vi "Set Up Dialog - Goniometer .vi"() -> ()   [LabVIEW 2012]
panel:
  out "Calibration Instructions":string="1. Connect the sensor to your myDAQ as shown in the diagram above.\n\n2. Use a text book to set the GNN-100 to an angle of 90°, type 90 for the SP1 Angle and record the voltage in SP1 Voltage.\n\n3. Set the GNN-100 straight, enter '0' for SP2 Angle, then record the voltage in SP2 Voltage."
  # "iWorx - Goniometer - Set Up"
  # "Goniometer (GNN - 100)"
  # "iWorx"
  # "Sensor"
  # "GNN - 100"
  # "myDAQ"
  # "Computer"
  # "Adaptor"
  # "Connection Diagram"
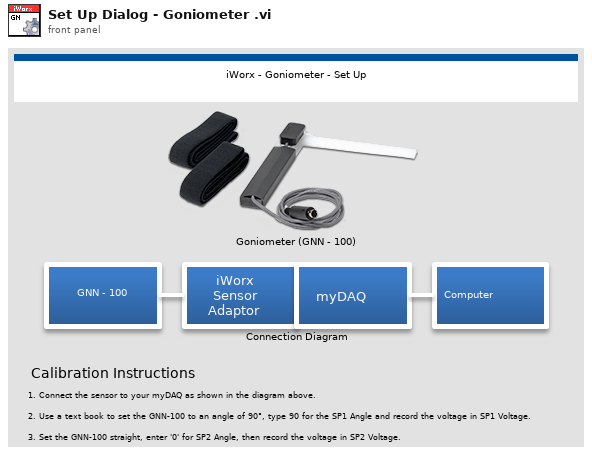
[diagram p1: front panel]
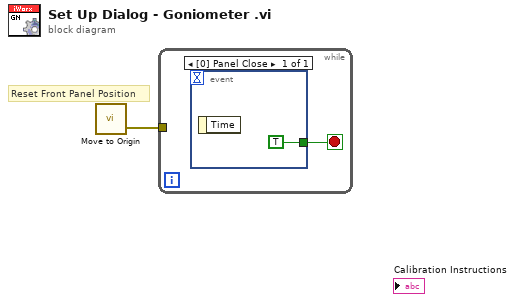
[diagram p0: block diagram]
diagram:
  # "Reset Front Panel Position"
  n1 = call "Move to Origin.vi"() -> ("Error Out"=w1:errorcluster)  [unwired: 3 in]
  n2 = while {
    tunnel: w1 -> [_]
    stop <- w2 stop-if-true
    n3 = event shown="[0] Panel Close" {
      selector: _ -> [_]
      dyn-events: _ -> [_]
      timeout: _ -> [_]
      tunnel: [TRUE] -> w2
      event Panel Close {
        n4 = event-data() -> ()  [unwired: 1 in, 1 out]
      }
    }
  }
